vi "get palette sections with items.vi"(8 "error in (no error)":errorcluster, 11 "nested palettes":T1(array[cluster])) -> (0 "error out":errorcluster, 3 "palette sections":T2(array[cluster]))   [LabVIEW 2020]
uses:
  <vilib>/xml/NI_XML.lvlib
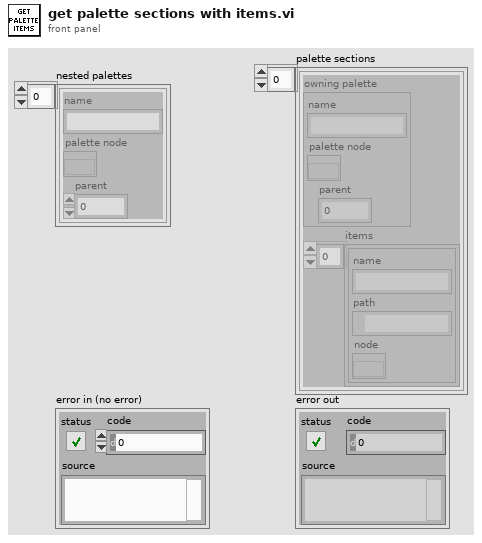
[diagram p1: front panel]
types:
  T1 = cluster{"name":string, "palette node":refnum<k20>, "parent":i32}[]
  T2 = cluster{"owning palette":cluster{"name":string, "palette node":refnum<k20>, "parent":i32}, "items":cluster{"name":string, "path":path, "node":refnum<k20>}[]}[]
  T3 = cluster{"node text":string, path, "node out":refnum<k20>}
  T4 = cluster{cluster{"name":string, "palette node":refnum<k20>, "parent":i32}, cluster{"node text":string, path, "node out":refnum<k20>}[]}
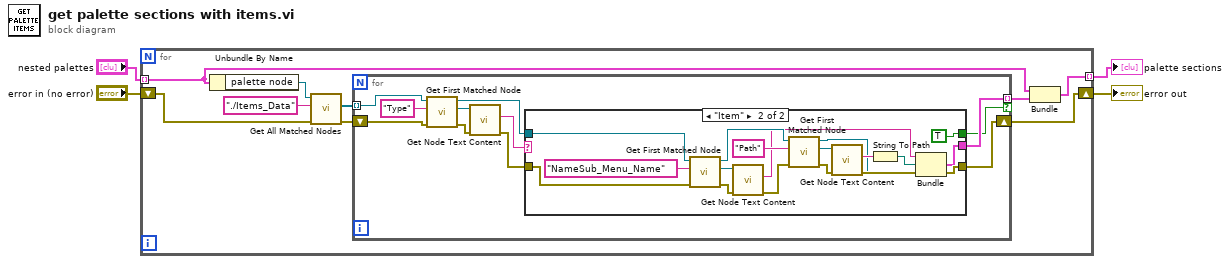
[diagram p0: block diagram]
diagram:
  n1 = for {
    shift-right: [w8] -> w2
    shift-left: "error in (no error)" -> [w12]
    tunnel: "nested palettes" -> [w7] mode=indexing
    tunnel: [w5] -> w4 mode=indexing
    n2 = Unbundle By Name(w7) -> ("palette node"=w13:refnum<k20>)
    n3 = call <vilib>:"Get All Matched Nodes.vi"("error in (no error)"=w12, "XPath expression"="./Items_Data", "node in"=w13) -> ("error out"=w11:errorcluster, "node result array"=w9:refnum<k20>[])  [unwired: 6 in, 1 out]
    n4 = for {
      tunnel: w9 -> [w22] mode=indexing
      shift-right: [w17] -> w8
      shift-left: w11 -> [w24]
      tunnel: [w15] -> w6 mode=indexing if=w14
      n5 = call <vilib>:"Get First Matched Node.vi"("error in (no error)"=w24, "XPath expression"="Type", "node in"=w22) -> ("error out"=w23:errorcluster, "node result"=w18:refnum<k20>, "node out"=w21:refnum<k20>)  [unwired: 6 in]
      n6 = call <vilib>:"Get Node Text Content.vi"("error in (no error)"=w23, "node in"=w18) -> ("error out"=w19:errorcluster, "node text"=w16:string)  [unwired: 7 in, 1 out]
      n7 = case shown="\"Item\"" w16 {
        tunnel: w21 -> [_ w38]
        tunnel: w19 -> [w25 w37]
        tunnel: [w25 w32] -> w17
        tunnel: [_ w29] -> w15
        tunnel: [_ TRUE] -> w14
        frame Default {
        }
        frame "Item" {
          n8 = call <vilib>:"Get First Matched Node.vi"("error in (no error)"=w37, "XPath expression"="NameSub_Menu_Name", "node in"=w38) -> ("error out"=w40:errorcluster, "node result"=w33:refnum<k20>, "node out"=w42:refnum<k20>)  [unwired: 6 in]
          n9 = call <vilib>:"Get Node Text Content.vi"("error in (no error)"=w40, "node in"=w33) -> ("error out"=w34:errorcluster, "node text"=w30:string)  [unwired: 7 in, 1 out]
          n10 = call <vilib>:"Get First Matched Node.vi"("error in (no error)"=w34, "XPath expression"="Path", "node in"=w42) -> ("error out"=w36:errorcluster, "node result"=w35:refnum<k20>, "node out"=w26:refnum<k20>)  [unwired: 6 in]
          n11 = call <vilib>:"Get Node Text Content.vi"("error in (no error)"=w36, "node in"=w35) -> ("error out"=w32:errorcluster, "node text"=w31:string)  [unwired: 7 in, 1 out]
          n12 = String To Path(string=w31) -> (path=w27:path)
          n13 = Bundle("node text"=w30, w27, "node out"=w26) -> (w29:T3)  [unwired: 1 in]
        }
      }
    }
    n14 = Bundle(w7, w6) -> (w5:T4)  [unwired: 1 in]
  }
  "palette sections" <- w4
  "error out" <- w2
